vi "Keithley 2200 Series Output List File Settings.vi"() -> ()   [LabVIEW 2021]
doc: "DESCRIPTION:\n\nIn this VI commands executed in a certain order to successfully complete a list file. \n\nINSTRUCTIONS:\n1. Enter the resource name.\n2. Set a list in continuous or step mode with command order.\n3. Sets the voltage or current step. \n4. Sets the step time.\n5. Select Save or Recall operation ,to save or recall list file to or from memory \n6. Enter Non -volatile memory address, that the settings will be saved to. \n7. Configures the power supply for command List mode\n8. Run the VI.\n\nNOTES:\n\nNotice the order of the power supply component VIs in the block diagram. The first VI in a sequence is the power supply Initialize.vi, which provides a VISA session to the instrument driver. The last VI in a sequence must be the power supply Close.vi which closes the Visa session."
uses:
  <instrlib>/Keithley 2200 Series/Keithley 2200 Series.lvlib
panel:
  in  "Unit(V)":u16(ring) items=["V", "mV", "A", "mA"]
  in  "Enable Output (T: Enable)":bool=TRUE
  in  "Steps Count(2)":dbl=2.0
  in  "Step Time(1)":dbl=1.0
  in  "VISA resource name":refnum<visa-resource-name>
  in  "Memory Address(1)":dbl=1.0
  in  "List Name":string
  in  "List Unit(0:Second)":u16(ring) items=["Second", "Msecond"]
  in  "Manual Range(0.00)":dbl format="%.2f"
  in  "Number of Steps(1)":dbl=1.0 format="%.2f"
  in  "List Operation(0:Voltage)":u16(ring) items=["Voltage", "Current"]
  in  "List Repeat Mode(0:Once)":u16(ring) items=["Once", "Repeat  "]
  in  "List Mode(0:Continuous)":u16(ring) items=["Continuous", "Step"]
  # "(c) Copyright 2012 Keithley Instruments Inc  ALL RIGHTS RESERVED."
  # "Configure Mode"
  # "Configure List Operation"
  # "Configure Time"
  # "Save List File"
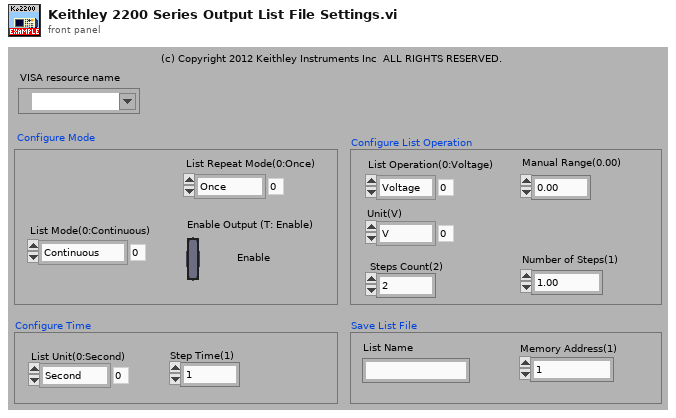
[diagram p1: front panel]
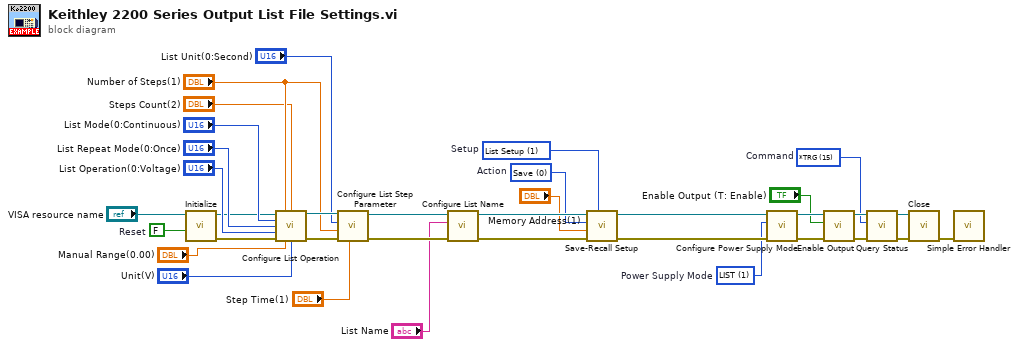
[diagram p0: block diagram]
diagram:
  w2 = u16 1 items=["Instrument Setup", "List Setup"]  # Setup
  w6 = u16 15 items=["*CLS", "*ESE", "*ESE?", "*RST", "*SRE", "*SRE?", "*STB?", "*ESR?", "*IDN?", "*OPC", "*OPC?", "*PSC", "*PSC?", "*SAV", "*RCL", "*TRG", "System Address", "Output State", "Output-Timer", "Output-Timer-State", "Digital Input Port- State", "Digital Output Port- State"]  # Command
  w18 = u16 1 items=["FIX", "LIST", "Digital milliohm meter "]  # Power Supply Mode
  w20 = u16 0 items=["Save", "Recall"]  # Action
  w35 = FALSE  # Reset
  n1 = call <instrlib>:"Initialize.vi"("Reset (True)"=w35, "VISA resource name"="VISA resource name") -> ("error out"=w4:errorcluster, "VISA resource name out"=w3:refnum<visa-resource-name>)  [unwired: 3 in, 5 out]
  n2 = call <instrlib>:"Configure List Operation.vi"("VISA resource name"=w3, "Number of Steps(1)"="Number of Steps(1)", "Steps Count(2)"="Steps Count(2)", "List Mode(0:Continuous)"="List Mode(0:Continuous)", "List Repeat Mode(0:Once)"="List Repeat Mode(0:Once)", "List Operation(0:Voltage)"="List Operation(0:Voltage)", "error in (no error)"=w4, "Manual Range(0.00)"="Manual Range(0.00)", "Unit(V)"="Unit(V)") -> ("VISA resource name out"=w34:refnum<visa-resource-name>, "error out"=w33:errorcluster)  [unwired: 5 out]
  n3 = call <instrlib>:"Configure List Step Parameter.vi"("Step Time(1)"="Step Time(1)", "error in (no error)"=w33, "List Step Number(2)"="Number of Steps(1)", "Unit(S)"="List Unit(0:Second)", "VISA resource name"=w34) -> ("error out"=w31:errorcluster, "VISA resource name out"=w32:refnum<visa-resource-name>)  [unwired: 5 out]
  n4 = call <instrlib>:"Configure List Name.vi"("error in (no error)"=w31, "List Name"="List Name", "VISA resource name"=w32) -> ("error out"=w29:errorcluster, "VISA resource name out"=w30:refnum<visa-resource-name>)  [unwired: 7 out]
  n5 = call <instrlib>:"Save-Recall Setup.vi"("Setup(0:Instrument Setup)"=w2, "error in (no error)"=w29, "Memory Address(1)"="Memory Address(1)", "Action(0:Save)"=w20, "VISA resource name"=w30) -> ("error out"=w27:errorcluster, "VISA resource name out"=w28:refnum<visa-resource-name>)  [unwired: 5 out]
  n6 = call <instrlib>:"Configure Power Supply Mode.vi"("error in (no error)"=w27, "Power Supply Mode (0:Fix)"=w18, "VISA resource name"=w28) -> ("error out"=w11:errorcluster, "VISA resource name out"=w12:refnum<visa-resource-name>)  [unwired: 7 out]
  n7 = call <instrlib>:"Enable Output.vi"("error in (no error)"=w11, "Enable Output (T: Enable)"="Enable Output (T: Enable)", "VISA resource name"=w12) -> ("error out"=w9:errorcluster, "VISA resource name out"=w10:refnum<visa-resource-name>)  [unwired: 7 out]
  n8 = call <instrlib>:"Query Status.vi"("error in (no error)"=w9, "Command (0:*CLS)"=w6, "VISA resource name"=w10) -> ("error out"=w7:errorcluster, "VISA resource name out"=w8:refnum<visa-resource-name>)  [unwired: 2 in, 5 out]
  n9 = call <instrlib>:"Close.vi"("error in (no error)"=w7, "VISA resource name"=w8) -> ("error out"=w16:errorcluster)  [unwired: 9 out]
  n10 = call <vilib>:"Simple Error Handler.vi"("error in (no error)"=w16) -> ()  [unwired: 1 in, 8 out]
